vi "poc.vi"(0 "TDATA":u64, 1 "reset":bool, 5 "TKEEP":u8, 7 "TVALID":bool, 9 "TLAST":bool, 11 "TUSER":bool) -> ()   [LabVIEW 2020]
uses:
  <instrlib>/_niInstr/Network/Types/v1/IPv4 Address.ctl
  <instrlib>/_niInstr/Network/Types/v1/MAC Address.ctl
  Ethernet MAC - Custom/Ethernet MAC - Custom.lvclass
  <instrlib>/_niInstr/Network/Ethernet/Utility/v1/FPGA/niInstr Ethernet Utilities FPGA v1.lvlib
  <instrlib>/_niInstr/Network/IPv4/FPGA/v1/niInstr IPv4 FPGA v1.lvlib
  <instrlib>/_niInstr/Network/IPv4/UDP/FPGA/v1/niInstr IPv4 UDP FPGA v1.lvlib
  <instrlib>/_niInstr/Network/Types/v1/niInstr Network Types v1.lvlib
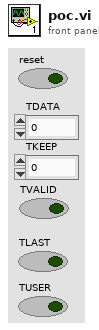
[diagram p1: front panel]
types:
  T1 = typedef "niInstr Network Types v1.lvlib/MAC Address.ctl" = u8[]
  T2 = typedef "niInstr Network Types v1.lvlib/IPv4 Address.ctl" = u8[]
  T3 = cluster{"TDATA":u64, "TKEEP":u8, "TVALID":bool, "TLAST":bool, "TUSER":bool}
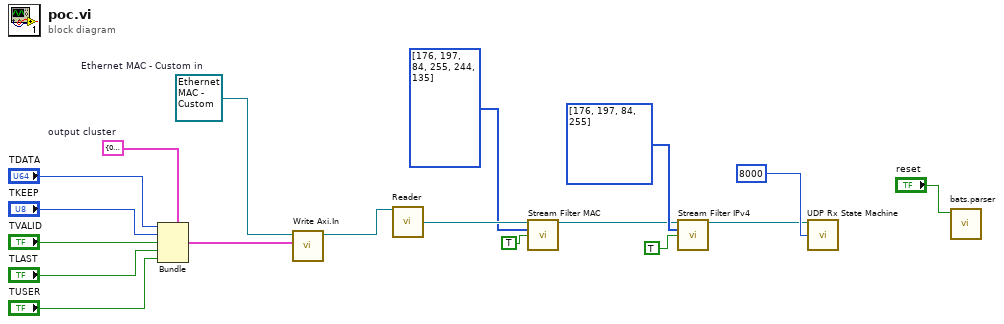
[diagram p0: block diagram]
diagram:
  w1 = refnum<class "Ethernet MAC - Custom.lvclass"> refnum  # Ethernet MAC - Custom in
  w14 = T3 {"TDATA"=0, "TKEEP"=0, "TVALID"=FALSE, "TLAST"=FALSE, "TUSER"=FALSE}  # output cluster
  n1 = Bundle(cluster=w14, "TDATA"="TDATA", "TKEEP"="TKEEP", "TVALID"="TVALID", "TLAST"="TLAST", "TUSER"="TUSER") -> (w10:T3)
  n2 = call-dynamic "Write Axi.In.vi"("Axi.In"=w10, "Ethernet MAC - Custom in"=w1) -> ("Ethernet MAC - Custom out"=w11:refnum<class "Ethernet MAC - Custom.lvclass">)  [unwired: 8 in, 1 out]
  n3 = call-dynamic "Reader.vi"("Ethernet MAC - Custom.lvclass"=w11) -> ("niInstr Ethernet MAC Raw Stream v1.lvclass"=w12:refnum<class "niInstr Ethernet MAC Raw Stream v1.lvclass">)  [unwired: 13 in, 1 out]
  n4 = call <instrlib>:"Stream Filter MAC.vi"("niInstr Ethernet MAC Raw Stream v1 in"=w12, "MAC Address"=T1 [176, 197, 84, 255, 244, 135], "Promiscuous?"=TRUE) -> ("niInstr Ethernet MAC Data Stream v1 out"=w3:refnum<class "niInstr Ethernet MAC Data Stream v1.lvclass">)  [unwired: 12 in]
  n5 = call <instrlib>:"Stream Filter IPv4.vi"("niInstr Ethernet MAC Data Stream v1 in"=w3, "IP Address"=T2 [176, 197, 84, 255], "disable IP filtering"=TRUE) -> ("niInstr IPv4 Data Stream out"=w2:refnum<class "niInstr IPv4 Data Stream v1.lvclass">)  [unwired: 12 in]
  n6 = call <instrlib>:"UDP Rx State Machine.vi"("niInstr IPv4 Data Stream in"=w2, "Dest Port"=u16 8000) -> ()  [unwired: 13 in, 1 out]
  n7 = call "bats.parser.vi"("reset"="reset") -> ()  [unwired: 10 in, 1 out]
